vi "Release.vi"(11 "Promise in":refnum<class "Promise.lvclass">) -> ()   [LabVIEW 2020, in "Promises.lvlib" / "Promise.lvclass"]
uses:
  Promise.lvclass
  Promise.lvclass/Promise.ctl
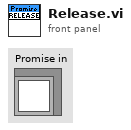
[diagram p1: front panel]
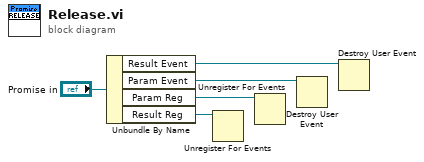
[diagram p0: block diagram]
diagram:
  n1 = Unbundle By Name("Promise in") -> ("Result Event"=w4:refnum<user-event>, "Param Event"=w3:refnum<user-event>, "Param Reg"=w2:refnum<event-registration>, "Result Reg"=w1:refnum<event-registration>)
  n2 = Unregister For Events(event registration refnum=w1) -> ()  [unwired: 1 in, 1 out]
  n3 = Unregister For Events(event registration refnum=w2) -> ()  [unwired: 1 in, 1 out]
  n4 = Destroy User Event(user event=w3) -> ()  [unwired: 1 in, 1 out]
  n5 = Destroy User Event(user event=w4) -> ()  [unwired: 1 in, 1 out]
